vi "Use_AppBuilder_Cache.vi"(8 "error in (no error)":errorcluster, 11 "AB_DLL in":refnum<class "AB_DLL.lvclass">) -> (0 "error out":errorcluster, 2 "use cache":bool, 3 "AB_DLL out":refnum<class "AB_DLL.lvclass">)   [LabVIEW 2020, in "AB_DLL.lvclass"]
uses:
  <vilib>/AppBuilder/AB_Classes/DLL/AB_DLL.lvclass
  e:/builds/penguin/labview/branches/2020/dev/dist/vi.lib/AppBuilder/AB_Classes/TargetFile/AB_Targetfile.lvclass
  <vilib>/AppBuilder/AB_Classes/TargetFile/AB_Targetfile.lvclass
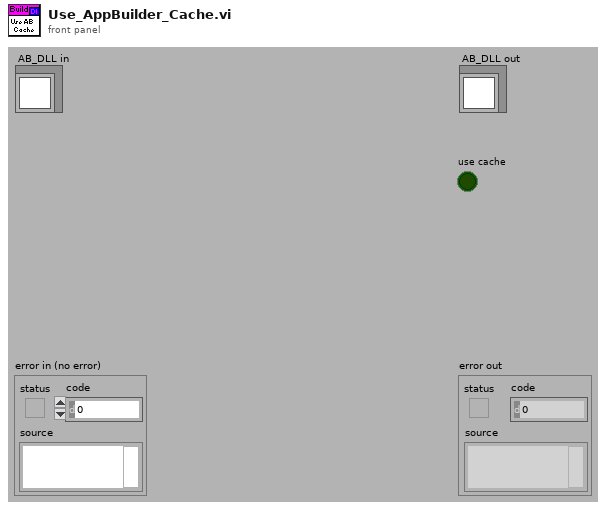
[diagram p1: front panel]
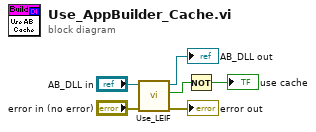
[diagram p0: block diagram]
diagram:
  n1 = call <vilib>:"Use_LEIF.vi"("error in (no error)"="error in (no error)", "AB_Targetfile in"="AB_DLL in") -> ("error out"=→"error out":errorcluster, "use LEIF?"=w3:bool, "AB_Targetfile out"=→"AB_DLL out":refnum<class "AB_DLL.lvclass">)  [unwired: 7 in]
  n2 = Not(x=w3) -> (.not. x?=→"use cache":bool)
